vi "FPGAsubPulse.vi"(1 "Signal Sign":bool=TRUE, 2 "Signal start":u64, 3 "Signal stop":u64, 4 "Clock":u64) -> (0 "Boolean":bool)   [LabVIEW 2009]
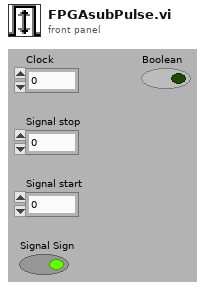
[diagram p1: front panel]
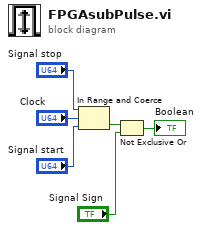
[diagram p0: block diagram]
diagram:
  n1 = In Range and Coerce(upper limit="Signal stop", x="Clock", lower limit="Signal start") -> (In Range?=w5:bool)  [unwired: 1 out]
  n2 = Not Exclusive Or(1:"Signal Sign", 2:w5) -> (0:→"Boolean":bool)
